vi "AES Encryption Example Using Classes.vi"() -> ()   [LabVIEW 2016]
uses:
  Crypto.AES/Crypto.AES.lvclass
panel:
  out "Encoded Data":string
  out "data":errorcluster
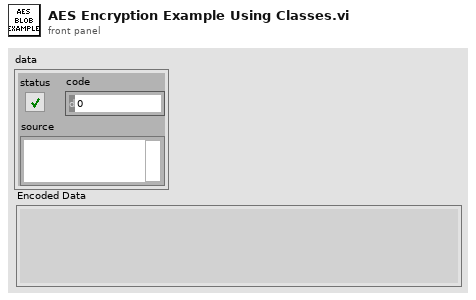
[diagram p1: front panel]
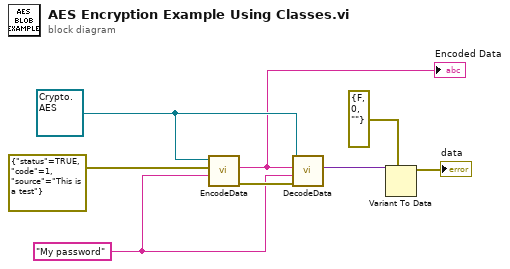
[diagram p0: block diagram]
diagram:
  w4 = "My password" ("Secret")
  w6 = refnum<class "Crypto.AES.lvclass"> refnum ("Crypto.AES.lvclass")
  n1 = call-dynamic "EncodeData.vi"("Secret"=w4, "Data to Encode"=errorcluster {"status"=TRUE, "code"=1, "source"="This is a test"} ("error in (no error)"), "CryptoType"=w6) -> ("error out"=w7:errorcluster, "Encoded Data"=w5:string)  [unwired: 7 in]
  "Encoded Data" <- w5
  n2 = call-dynamic "DecodeData.vi"("error in (no error)"=w7, "Secret"=w4, "Encoded Data"=w5, "CryptoType"=w6) -> ("Decoded Data"=w3:variant)  [unwired: 6 in, 1 out]
  n3 = Variant To Data(type=errorcluster {"status"=FALSE, "code"=0, "source"=""} ("error out"), Variant=w3) -> (data=→"data":errorcluster)  [unwired: 1 in, 1 out]
